vi "MH_CalcDeltaT.vi"(5 "Buffsize":i32, 6 "WinIndex":i32, 7 "TrueTime":u64, 9 "WIndowW":i32, 10 "Data In":u64[](array[numeric]), 11 "Buffindex":i32) -> (1 "WinIndexOut":i32, 2 "NewDelta":bool, 3 "DeltaT Out":i32[](array[numeric]))   [LabVIEW 2019]
panel:
  # "here"
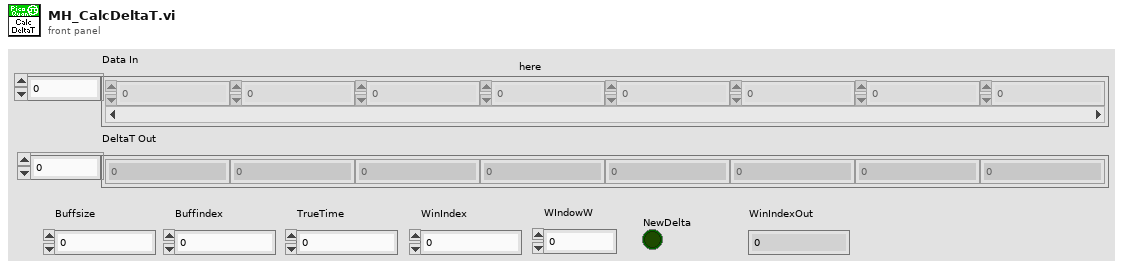
[diagram p1: front panel]
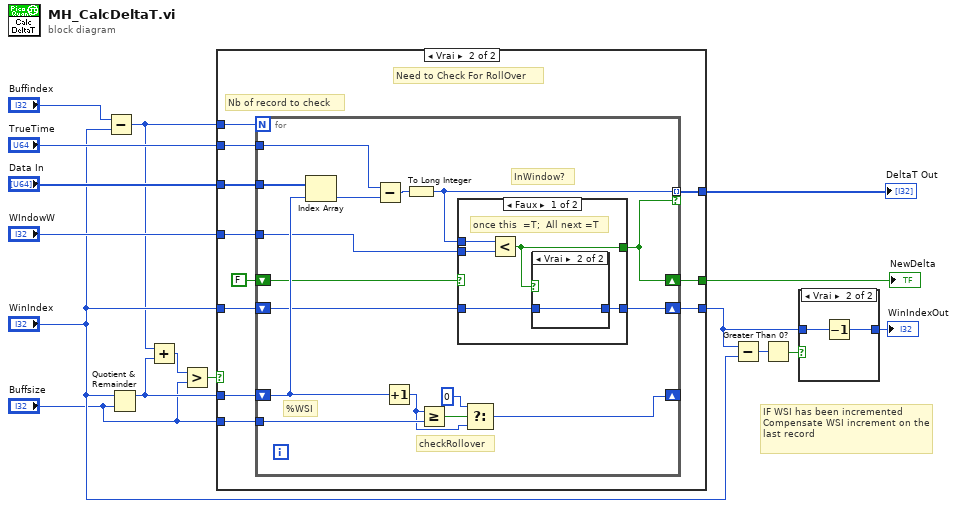
[diagram p0: block diagram]
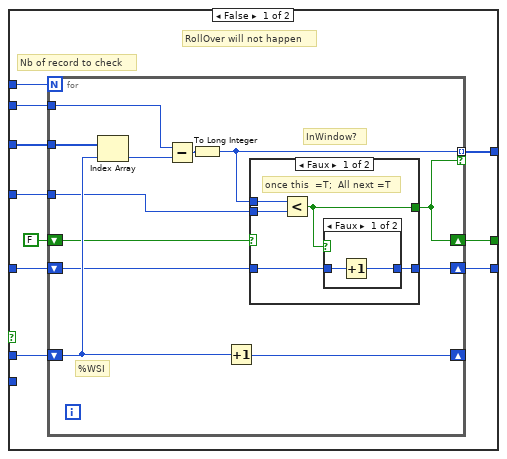
[diagram p2: hidden frame]
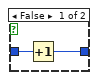
[diagram p5: hidden frame]
diagram:
  # "IF WSI has been incremented\nCompensate WSI increment on the last record"
  n1 = Subtract(x="Buffindex", y="WinIndex") -> (x-y=w5:i32)
  n2 = Quotient & Remainder(x="WinIndex", y="Buffsize") -> (x-y*floor(x/y)=w4:i32)  [unwired: 1 out]
  n3 = Add(x=w5, y=w4) -> (x+y=w3:i32)
  n4 = Greater?(x=w3, y="Buffsize") -> (0:w1:bool)
  n5 = case shown="Vrai" w1 {
    tunnel: "Data In" -> [w26 w59]
    tunnel: "TrueTime" -> [w25 w58]
    tunnel: "WIndowW" -> [w24 w57]
    tunnel: [w23 w49] -> w12
    tunnel: [w22 w56] -> w11
    tunnel: "WinIndex" -> [w20 w54]
    tunnel: [w19 w53] -> w6
    tunnel: w5 -> [w18 w52]
    tunnel: w4 -> [w17 w51]
    tunnel: "Buffsize" -> [_ w50]
    frame False {
      # "RollOver will not happen"
      # "Nb of record to check"
      n6 = for {
        N: w18 -> [_]
        tunnel: w26 -> [w36]
        tunnel: w25 -> [w38]
        tunnel: [w37] -> w23 mode=indexing if=w31
        shift-right: [w28] -> w19
        shift-left: w20 -> [w29]
        shift-right: [w27] -> _
        shift-left: w17 -> [w33]
        tunnel: w24 -> [w32]
        shift-right: [w31] -> w22
        shift-left: FALSE -> [w30]
        # "InWindow?"
        # "%WSI"
        n7 = Index Array(array=w36, index=w33) -> (element=w34:u64)
        n8 = Subtract(x=w38, y=w34) -> (x-y=w35:u64)
        n9 = To Long Integer(number=w35) -> (32bit integer=w37:i32)
        n10 = Increment(x=w33) -> (x+1=w27:i32)
        n11 = case shown="Faux" w30 {
          selector: w30 -> [_ w47]
          tunnel: w37 -> [w43 _]
          tunnel: w32 -> [w42 _]
          tunnel: [w39 w47] -> w31
          tunnel: w29 -> [w41 w48]
          tunnel: [w40 w48] -> w28
          frame False {
            # "once this  =T;  All next =T"
            n12 = Less?(x=w43, y=w42) -> (x < y?=w39:bool)
            n13 = case shown="Faux" w39 {
              tunnel: w41 -> [w45 w46]
              tunnel: [w44 w46] -> w40
              frame False {
                n14 = Increment(x=w45) -> (x+1=w44:i32)
              }
              frame True {
              }
            }
          }
          frame True {
          }
        }
      }
    }
    frame True {
      # "Need to Check For RollOver"
      # "Nb of record to check"
      n15 = for {
        N: w52 -> [_]
        tunnel: w59 -> [w73]
        tunnel: w58 -> [w75]
        tunnel: [w74] -> w49 mode=indexing if=w66
        shift-right: [w63] -> w53
        shift-left: w54 -> [w64]
        shift-right: [w68] -> _
        shift-left: w51 -> [w69]
        tunnel: w50 -> [w70]
        tunnel: w57 -> [w67]
        shift-right: [w66] -> w56
        shift-left: FALSE -> [w65]
        # "checkRollover"
        # "InWindow?"
        # "%WSI"
        n16 = Index Array(array=w73, index=w69) -> (element=w71:u64)
        n17 = Subtract(x=w75, y=w71) -> (x-y=w72:u64)
        n18 = Increment(x=w69) -> (x+1=w60:i32)
        n19 = To Long Integer(number=w72) -> (32bit integer=w74:i32)
        n20 = Greater Or Equal?(x=w60, y=w70) -> (x >= y?=w62:bool)
        n21 = case shown="Faux" w65 {
          selector: w65 -> [_ w84]
          tunnel: w74 -> [w80 _]
          tunnel: w67 -> [w79 _]
          tunnel: [w76 w84] -> w66
          tunnel: w64 -> [w78 w85]
          tunnel: [w77 w85] -> w63
          frame False {
            # "once this  =T;  All next =T"
            n22 = Less?(x=w80, y=w79) -> (x < y?=w76:bool)
            n23 = case shown="Vrai" w76 {
              tunnel: w78 -> [w82 w83]
              tunnel: [w81 w83] -> w77
              frame False {
                n24 = Increment(x=w82) -> (x+1=w81:i32)
              }
              frame True {
              }
            }
          }
          frame True {
          }
        }
        n25 = Select(t=0 ("x+1"), s=w62, f=w60) -> (s? t:f=w68:i32)
      }
    }
  }
  "DeltaT Out" <- w12
  "NewDelta" <- w11
  n26 = Subtract(x=w6, y="WinIndex") -> (x-y=w9:i32)
  n27 = Greater Than 0?(x=w9) -> (x > 0?=w8:bool)
  n28 = case shown="Vrai" w8 {
    tunnel: [w86 w87] -> w7
    tunnel: w6 -> [w86 w88]
    frame False {
    }
    frame True {
      n29 = Decrement(x=w88) -> (x-1=w87:i32)
    }
  }
  "WinIndexOut" <- w7
